vi "Create PID wrapper.vi"(1 "D":dbl, 2 "I":dbl, 3 "P":dbl) -> (0 "PIDClass string":string)   [LabVIEW 2011]
uses:
  PIDClass.lvclass
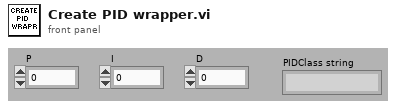
[diagram p1: front panel]
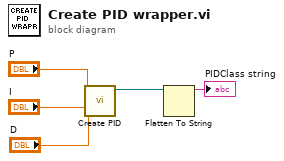
[diagram p0: block diagram]
diagram:
  n1 = call "Create PID.vi"("D"="D", "I"="I", "P"="P") -> ("PIDClass.lvclass"=w2:refnum<class "PIDClass.lvclass">)  [unwired: 8 out]
  n2 = Flatten To String(anything=w2) -> (data string=→"PIDClass string":string)  [unwired: 1 in, 4 out]
